vi "NI VeriStand - Get Channel 2D Array Values.vi"(8 "error in (no error)":errorcluster, 10 "Channel":string, 11 "WorkspaceManager in":T1) -> (0 "error out":errorcluster, 2 "Values":dbl[][](array[numeric]), 3 "WorkspaceManager out":T1)   [LabVIEW 2020, in "NI_VS Workspace ExecutionAPI.lvlib"]
doc: "Returns values of channels on the target. You can get values for a single channel, multiple channels, or vector values for a single channel. You must manually select the polymorphic instance to use."
uses:
  <vilib>/NI VeriStand/Execution/Workspace/NI_VS Workspace ExecutionAPI.lvlib
  <vilib>/NI VeriStand/Execution/Workspace/WorkspaceAPI.ctl
  NationalInstruments.VeriStand.ClientAPI
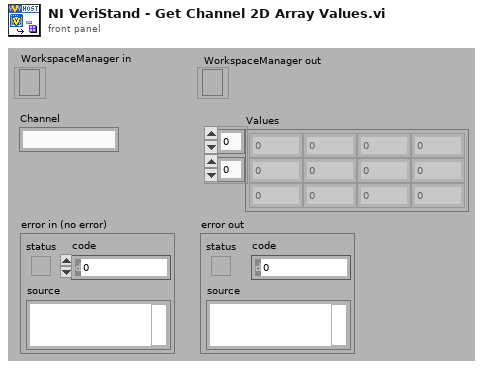
[diagram p1: front panel]
types:
  T1 = typedef "NI_VS Workspace ExecutionAPI.lvlib/WorkspaceAPI.ctl" = refnum<k24>
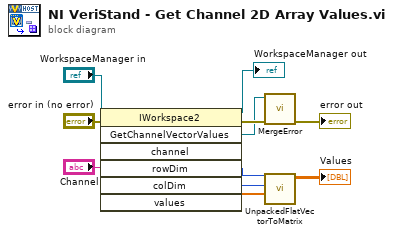
[diagram p0: block diagram]
diagram:
  n1 = invoke class="IWorkspace2" method="GetChannelVectorValues"(reference="WorkspaceManager in", error in="error in (no error)", "channel"="Channel") -> (reference out=→"WorkspaceManager out":T1, error out=w9:errorcluster, "GetChannelVectorValues"=w1:refnum<k24>, "rowDim"=w5:u32, "colDim"=w4:u32, "values"=w3:dbl[])  [unwired: 4 in, 1 out]
  n2 = call <vilib>:"MergeError.vi"("error in (no error)"=w9, "Error"=w1) -> ("error out"=→"error out":errorcluster)  [unwired: 9 out]
  n3 = call <vilib>:"UnpackedFlatVectorToMatrix.vi"("FlatValues"=w3, "colDim"=w4, "rowDim"=w5) -> ("Matrix"=→"Values":dbl[][])  [unwired: 8 out]
